vi "ReadBlock.vi"(0 "VISA Refnum in":refnum<visa-resource-name>, 3 "error in (no error)":errorcluster) -> (7 "VISA Refnum out":refnum<visa-resource-name>, 8 "Temperature":dbl, 10 "error out":errorcluster)   [LabVIEW 2023]
uses:
  <vilib>/Utility/error.llb/Error Cluster From Error Code.vi
  <vilib>/regexp/Match Regular Expression.xnode
  <vilib>/ErrorRing/Error Ring.xnode
panel:
  out "String":string
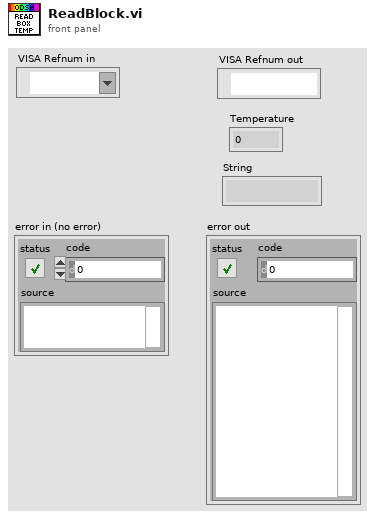
[diagram p1: front panel]
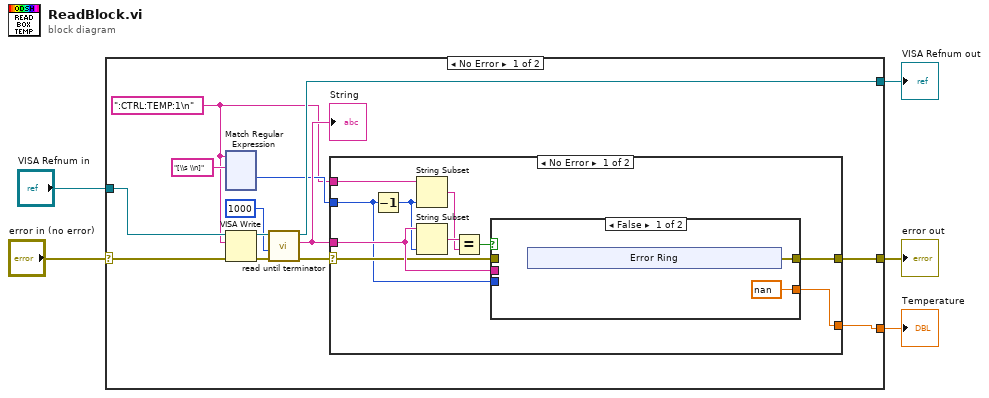
[diagram p0: block diagram]
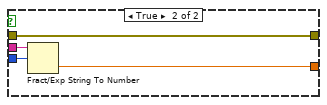
[diagram p2: hidden frame]
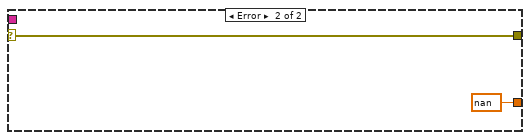
[diagram p3: hidden frame]
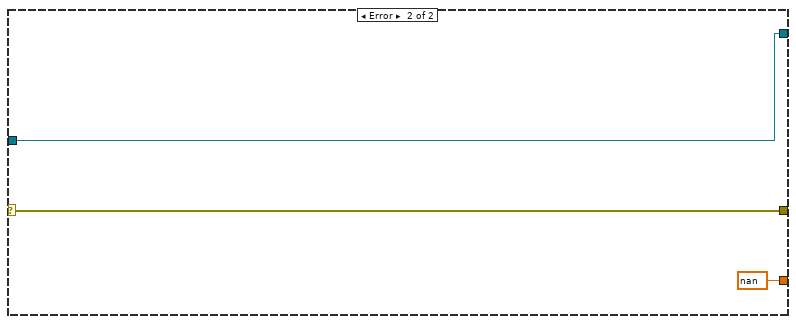
[diagram p4: hidden frame]
diagram:
  n1 = case shown="No Error" "error in (no error)" {
    selector: "error in (no error)" -> [w6 w161]
    tunnel: "VISA Refnum in" -> [w18 w160]
    tunnel: [w15 w160] -> w4
    tunnel: [w13 nan] -> w3
    tunnel: [w11 w161] -> w2
    frame No Error {
      w7 = ":CTRL:TEMP:1\n" ("buffer d'écriture")
      n2 = xnode "Match Regular Expression"("chaîne en entrée"=w7, "expression régulière"="[\\s \\n]" ("regular expression")) -> ("offset après correspondance"=w8:i32)  [unwired: 4 in, 4 out]
      n3 = VISA Write(VISA resource name=w18, write buffer=w7, error in (no error)=w6) -> (VISA resource name out=w17:refnum<visa-resource-name>, error out=w16:errorcluster)  [unwired: 1 out]
      n4 = call "read until terminator.vi"("error in (no error)"=w16, "Timeout (ms)"=1000, "VISA Refnum in"=w17) -> ("error out"=w12:errorcluster, "String"=w10:string, "VISA Refnum out"=w15:refnum<visa-resource-name>)  [unwired: 6 in]
      "String" <- w10
      n5 = case shown="No Error" w12 {
        selector: w12 -> [w139 w157]
        tunnel: w10 -> [w143 _]
        tunnel: [w145 nan] -> w13
        tunnel: [w138 w157] -> w11
        tunnel: w8 -> [w137 _]
        tunnel: w7 -> [w144 _]
        frame No Error {
          n6 = Decrement(x=w137) -> (x-1=w136:i32)
          n7 = String Subset(string=w144, length (rest)=w136) -> (substring=w141:string)  [unwired: 1 in]
          n8 = String Subset(string=w143, length (rest)=w136) -> (substring=w142:string)  [unwired: 1 in]
          n9 = Equal?(x=w142, y=w141) -> (x = y?=w140:bool)
          n10 = case shown="False" w140 {
            tunnel: [nan w156] -> w145
            tunnel: w143 -> [_ w155]
            tunnel: w137 -> [_ w154]
            tunnel: w139 -> [_ w153]
            tunnel: [w146 w153] -> w138
            frame False {
              n11 = xnode "Error Ring"() -> ("error out"=w146:errorcluster)
            }
            frame True {
              n12 = Fract/Exp String To Number(string=w155, offset=w154) -> (number=w156:dbl)  [unwired: 2 in, 1 out]
            }
          }
        }
        frame Error {
        }
      }
    }
    frame Error {
    }
  }
  "error out" <- w2
  "VISA Refnum out" <- w4
  "Temperature" <- w3
